vi "Write 1D Array I8.vi"(8 "error in (no error)":errorcluster, 9 "start index in (0)":i64, 10 "value":i8[](array[numeric]), 11 "pointer in":u64) -> (0 "error out":errorcluster, 1 "start index out":i64, 2 "number of elements":i64, 3 "pointer out":u64)   [LabVIEW 2013, in "Linux RT IPC.lvlib" / "Shared Memory.lvlib"]
uses:
  Shared Memory.lvlib
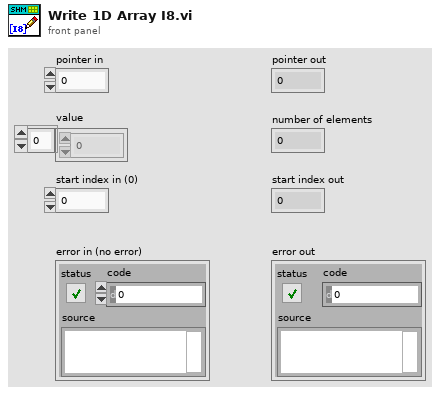
[diagram p1: front panel]
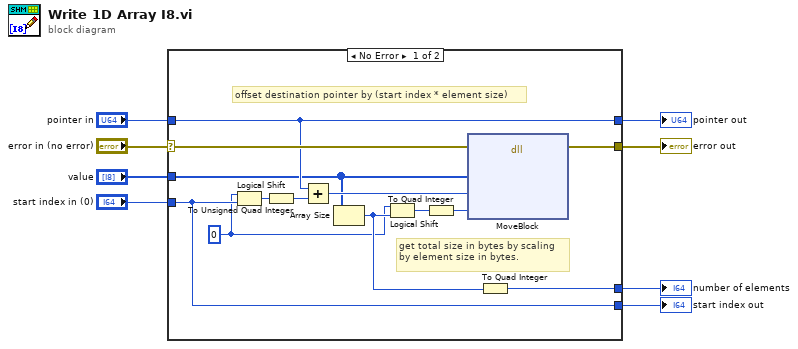
[diagram p0: block diagram]
diagram:
  n1 = case shown="No Error" "error in (no error)" {
    selector: "error in (no error)" -> [w17 w24]
    tunnel: [w16 w24] -> w8
    tunnel: "pointer in" -> [w14 w23]
    tunnel: "value" -> [w9 _]
    tunnel: [w14 w23] -> w5
    tunnel: [w10 _] -> w4
    tunnel: "start index in (0)" -> [w13 w22]
    tunnel: [w13 w22] -> w2
    frame No Error {
      w11 = i16 0 ("y")
      # "get total size in bytes by scaling by element size in bytes."
      # "offset destination pointer by (start index * element size)"
      n2 = Logical Shift(y=w11, x=w13) -> (x << y=w20:i64)
      n3 = To Unsigned Quad Integer(1:w20) -> (0:w21:u64)
      n4 = Add(x=w14, y=w21) -> (x+y=w15:u64)
      n5 = Array Size(array=w9) -> (size(s)=w12:i32)
      n6 = Logical Shift(y=w11, x=w12) -> (x << y=w19:i32)
      n7 = To Quad Integer(1:w19) -> (0:w18:i64)
      n8 = dll-call lib="LabVIEW" fn="MoveBlock"(error in=w17, "data"=w9, "pointer"=w15, "size"=w18) -> (error out=w16:errorcluster)  [unwired: 6 in, 1 out]
      n9 = To Quad Integer(1:w12) -> (0:w10:i64)
    }
    frame Error {
    }
  }
  "error out" <- w8
  "pointer out" <- w5
  "number of elements" <- w4
  "start index out" <- w2
